vi "Read Asynchronous Measurement (Voltage).vi"(6 "Wait Time (10 S)":i32=10, 7 "Voltage Buffer (smua.nvbuffer1)":string="smua.nvbuffer1", 8 "error in (no error)":errorcluster, 10 "Source Measure Unit Channel (0: Channel A)":i32(ring) items=["Channel A", "Channel B"], 11 "VISA resource name":refnum<visa-resource-name>) -> (0 "error out":errorcluster, 1 "Voltage Buffer Data (V)":dbl[](array[numeric]), 3 "VISA resource name out":refnum<visa-resource-name>)   [LabVIEW 2017, in "Keithley 2600 Series.lvlib"]
doc: "Returns the asynchronous voltage measurements."
uses:
  <instrlib>/Keithley 2600 Series/Keithley 2600 Series.lvlib
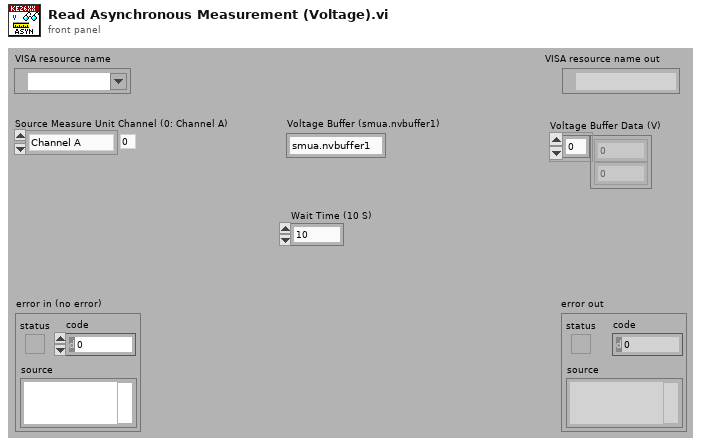
[diagram p1: front panel]
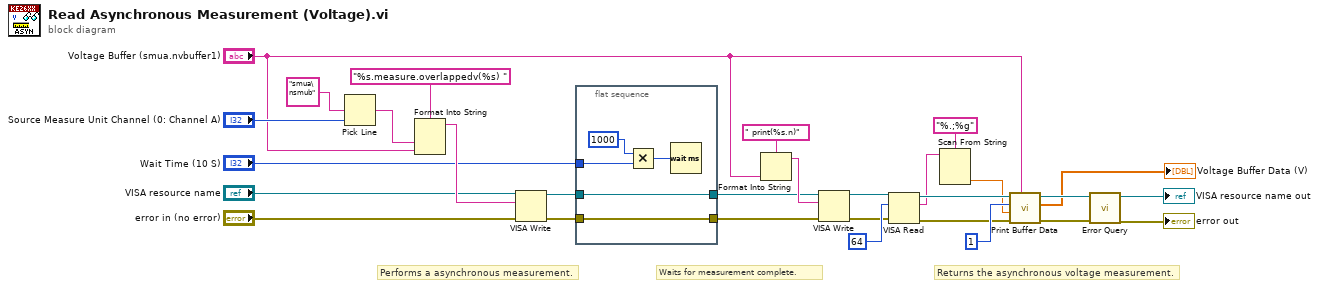
[diagram p0: block diagram]
diagram:
  # "Performs a asynchronous measurement."
  # "Waits for measurement complete."
  # "Returns the asynchronous voltage measurement."
  n1 = Pick Line(multi-line string="smua\nsmub", line index="Source Measure Unit Channel (0: Channel A)") -> (output string=w20:string)  [unwired: 1 in]
  n2 = Format Into String(format string="%s.measure.overlappedv(%s) ", w20, "Voltage Buffer (smua.nvbuffer1)") -> (resulting string=w26:string)  [unwired: 2 in, 1 out]
  n3 = VISA Write(VISA resource name="VISA resource name", write buffer=w26, error in (no error)="error in (no error)") -> (VISA resource name out=w7:refnum<visa-resource-name>, error out=w5:errorcluster)  [unwired: 1 out]
  n4 = flat-sequence {
    tunnel: "Wait Time (10 S)" -> [w34]
    tunnel: w7 -> [w31]
    tunnel: [w31] -> w6
    tunnel: w5 -> [w30]
    tunnel: [w30] -> w4
    frame #0 {
      n5 = Multiply(x=1000, y=w34) -> (x*y=w32:i32)
      n6 = Wait (ms)(milliseconds to wait=w32) -> ()  [unwired: 1 out]
    }
  }
  n7 = Format Into String(format string=" print(%s.n)", "Voltage Buffer (smua.nvbuffer1)") -> (resulting string=w9:string)  [unwired: 2 in, 1 out]
  n8 = VISA Write(VISA resource name=w6, write buffer=w9, error in (no error)=w4) -> (VISA resource name out=w3:refnum<visa-resource-name>, error out=w2:errorcluster)  [unwired: 1 out]
  n9 = VISA Read(VISA resource name=w3, byte count=u32 64, error in (no error)=w2) -> (VISA resource name out=w23:refnum<visa-resource-name>, read buffer=w19:string, error out=w22:errorcluster)  [unwired: 1 out]
  n10 = Scan From String(format string="%.;%g", input string=w19) -> (output 1=w18:dbl)  [unwired: 3 in, 3 out]
  n11 = call <instrlib>:"Print Buffer Data.vi"("Reading Buffer (smua.nvbuffer1)"="Voltage Buffer (smua.nvbuffer1)", "error in (no error)"=w22, "End Index (1)"=w18, "Start Index (1)"=1 ("Start Index (0)"), "VISA resource name"=w23) -> ("error out"=w16:errorcluster, "Buffer Data"=→"Voltage Buffer Data (V)":dbl[], "VISA resource name out"=w17:refnum<visa-resource-name>)  [unwired: 4 in]
  n12 = call <instrlib>:"Error Query.vi"("error in (no error)"=w16, "VISA resource name"=w17) -> ("error out"=→"error out":errorcluster, "VISA resource name out"=→"VISA resource name out":refnum<visa-resource-name>)  [unwired: 6 in, 2 out]
